vi "Query.vi"(8 "error in (no error)":errorcluster, 9 "Timeout":i32=10000, 10 "Query":string, 11 "Postgres Connector In":refnum<class "Postgres Connector.lvclass">) -> (0 "error out":errorcluster, 2 "Query Return":T1[](array[typedef]), 3 "Postgres Connector Out":refnum<class "Postgres Connector.lvclass">)   [LabVIEW 2020, in "Postgres Connector.lvclass"]
doc: "This VI is used to send a query and retrieve the answer from the PostgreSQL Database"
uses:
  Postgres Connector.lvclass
  Cluster_Return_Of_The_Query.ctl
  Postgres Connector.lvclass/Postgres Connector.ctl
panel:
  out "ReadyForQuery":string
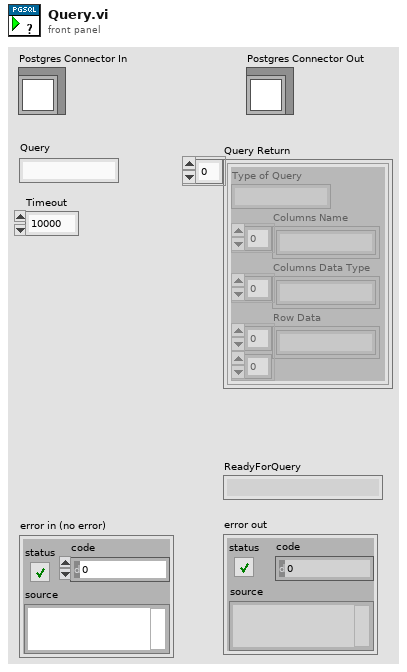
[diagram p1: front panel]
types:
  T1 = typedef "Postgres Connector.lvclass/Cluster_Return_Of_The_Query.ctl" = cluster{"Type of Query":string, "Columns Name":string[], "Columns Data Type":string[], "Row Data":string[][]}
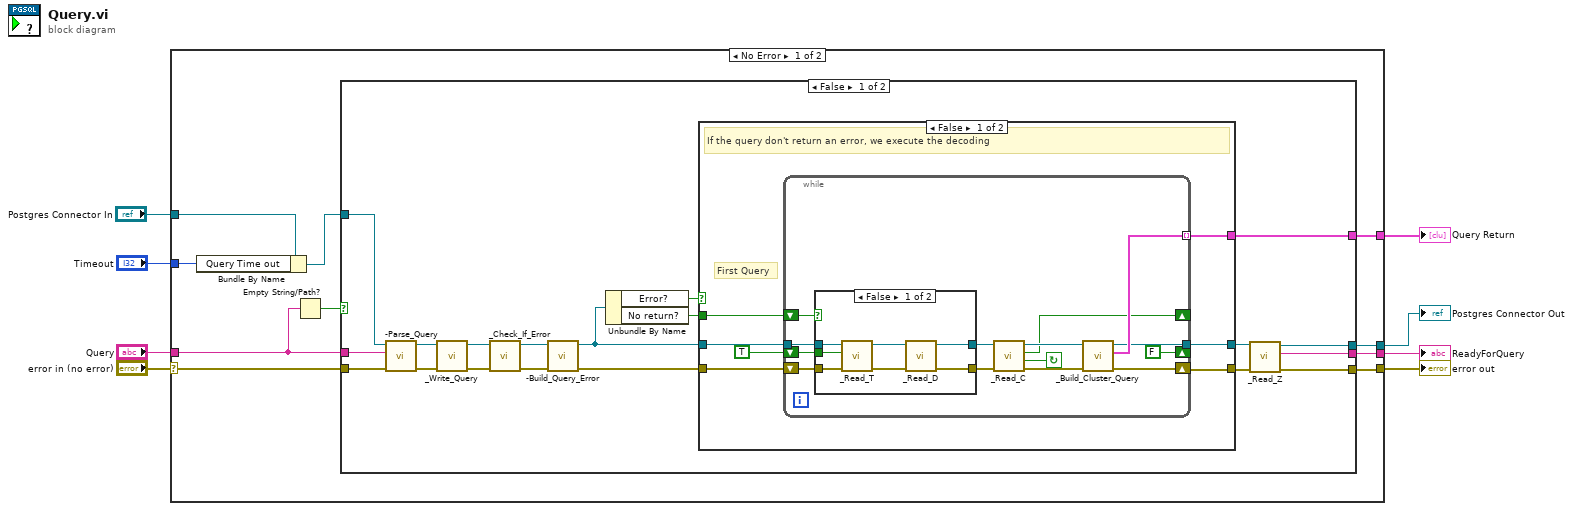
[diagram p0: block diagram]
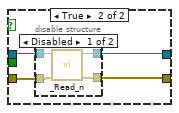
[diagram p2: hidden frame]
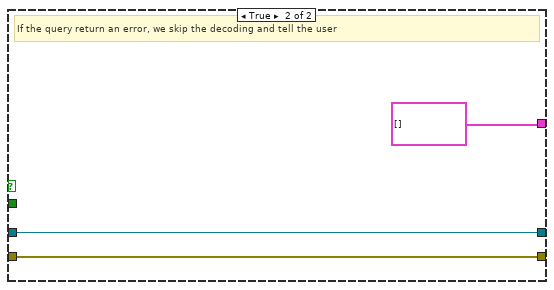
[diagram p4: hidden frame]
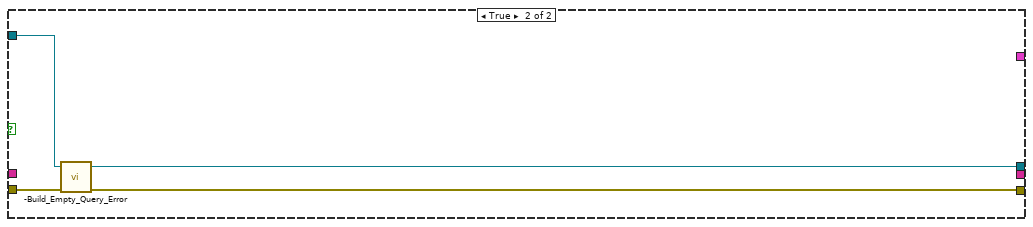
[diagram p5: hidden frame]
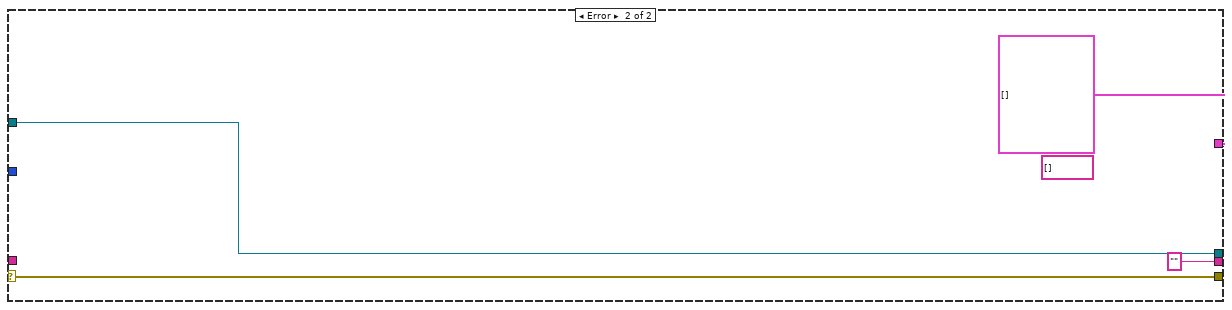
[diagram p6: hidden frame]
diagram:
  n1 = case shown="No Error" "error in (no error)" {
    selector: "error in (no error)" -> [w18 w84]
    tunnel: [w11 w84] -> w7
    tunnel: "Query" -> [w10 _]
    tunnel: "Postgres Connector In" -> [w14 w83]
    tunnel: [w15 w83] -> w5
    tunnel: [w16 "" ("ReadyForQuery")] -> w4
    tunnel: [w17 T1[] []] -> w3
    tunnel: "Timeout" -> [w13 _]
    frame No Error {
      n2 = Bundle By Name(cluster=w14, "Query Time out"=w13) -> (w12:refnum<class "Postgres Connector.lvclass">)
      n3 = Empty String/Path?(string/path=w10) -> (empty?=w9:bool)
      n4 = case shown="False" w9 {
        tunnel: w18 -> [w37 w79]
        tunnel: w10 -> [w36 _]
        tunnel: [w29 _] -> w17
        tunnel: [w28 _] -> w16
        tunnel: [w27 w80] -> w15
        tunnel: w12 -> [w22 w80]
        tunnel: [w21 w78] -> w11
        frame False {
          n5 = call "-Parse_Query.vi"("error in (no error)"=w37, "Query In"=w36, "Postgres Connector In"=w22) -> ("error out"=w35:errorcluster, "Postgres Connector Out"=w33:refnum<class "Postgres Connector.lvclass">)  [unwired: 7 in]
          n6 = call "_Write_Query.vi"("error in (no error)"=w35, "Postgres Connector In"=w33) -> ("error out"=w34:errorcluster, "Postgres Connector Out"=w20:refnum<class "Postgres Connector.lvclass">)  [unwired: 8 in]
          n7 = call "_Check_If_Error.vi"("error in (no error)"=w34, "Postgres Connector In"=w20) -> ("error out"=w26:errorcluster, "Postgres Connector Out"=w25:refnum<class "Postgres Connector.lvclass">)  [unwired: 8 in]
          n8 = call "-Build_Query_Error.vi"("error in (no error)"=w26, "Postgres Connector In"=w25) -> ("error out"=w24:errorcluster, "Postgres Connector Out"=w19:refnum<class "Postgres Connector.lvclass">)  [unwired: 8 in]
          n9 = Unbundle By Name(w19) -> ("Error?"=w31:bool, "No return?"=w23:bool)
          n10 = case shown="False" w31 {
            tunnel: [w40 w77] -> w32
            tunnel: w24 -> [w43 w77]
            tunnel: w19 -> [w42 w76]
            tunnel: [w41 w76] -> w30
            tunnel: [w39 T1[] []] -> w29
            tunnel: w23 -> [w38 _]
            frame False {
              # "First Query"
              # "If the query don't return an error, we execute the decoding"
              n11 = while {
                tunnel: w42 -> [w52]
                shift-right: [w57] -> w40
                shift-left: w43 -> [w56]
                shift-right: [FALSE] -> _
                shift-left: TRUE -> [w55]
                tunnel: [w45] -> w41
                tunnel: [w50] -> w39 mode=indexing
                shift-right: [w47] -> _
                shift-left: w38 -> [w48]
                stop <- w54 continue-if-true
                n12 = case shown="False" w48 {
                  tunnel: w56 -> [w63 w68]
                  tunnel: w55 -> [w62 _]
                  tunnel: w52 -> [w61 w65]
                  tunnel: [w59 w67] -> w46
                  tunnel: [w58 w66] -> w51
                  frame False {
                    n13 = call "_Read_T.vi"("error in (no error)"=w63, "First Query?"=w62, "Postgres Connector In"=w61) -> ("error out"=w64:errorcluster, "Postgres Connector Out"=w60:refnum<class "Postgres Connector.lvclass">)  [unwired: 7 in]
                    n14 = call "_Read_D.vi"("error in (no error)"=w64, "Postgres Connector In"=w60) -> ("error out"=w59:errorcluster, "Postgres Connector Out"=w58:refnum<class "Postgres Connector.lvclass">)  [unwired: 8 in]
                  }
                  frame True {
                    n15 = disable-structure shown="Disabled" {
                      disable-tunnel: w68 -> [w72 w73]
                      disable-tunnel: [w71 w73] -> w67
                      disable-tunnel: [w70 w74] -> w66
                      disable-tunnel: w65 -> [w69 w74]
                      frame Disabled {
                        n16 = call "_Read_n.vi"("error in (no error)"=w72, "Postgres Connector In"=w69) -> ("error out"=w71:errorcluster, "Postgres Connector Out"=w70:refnum<class "Postgres Connector.lvclass">)  [unwired: 7 in, 1 out]
                      }
                      frame Enabled {
                      }
                    }
                  }
                }
                n17 = call "_Read_C.vi"("error in (no error)"=w46, "Postgres Connector In"=w51) -> ("error out"=w57:errorcluster, "Another Query?"=w54:bool, "No return?"=w47:bool, "Postgres Connector Out"=w49:refnum<class "Postgres Connector.lvclass">)  [unwired: 6 in]
                n18 = call "_Build_Cluster_Query.vi"("Postgres Connector In"=w49) -> ("Query Return"=w50:T1, "Postgres Connector Out"=w45:refnum<class "Postgres Connector.lvclass">)  [unwired: 7 in, 2 out]
              }
            }
            frame True {
              # "If the query return an error, we skip the decoding and tell the user"
            }
          }
          n19 = call "_Read_Z.vi"("error in (no error)"=w32, "Postgres Connector In"=w30) -> ("error out"=w21:errorcluster, "State After Query"=w28:string, "Postgres Connector Out"=w27:refnum<class "Postgres Connector.lvclass">)  [unwired: 7 in]
        }
        frame True {
          n20 = call "-Build_Empty_Query_Error.vi"("error in (no error)"=w79) -> ("error out"=w78:errorcluster)  [unwired: 10 in]
        }
      }
    }
    frame Error {
      (unwired) string[] []
    }
  }
  "error out" <- w7
  "Postgres Connector Out" <- w5
  "ReadyForQuery" <- w4
  "Query Return" <- w3
